vi "Load UI Config.vi"(8 "error in (no error)":errorcluster, 10 "VariableName":string, 11 "MainName":string) -> (0 "error out":errorcluster, 1 "2D Array":string[][](array[string]), 3 "1D Array":string[](array[string]), 5 "new file path (Not A Path if cancelled)":path)   [LabVIEW 2021]
uses:
  <vilib>/Utility/file.llb/Read Delimited Spreadsheet (string).vi
  <userlib>/John_Lib/TopPath/TopPath.lvlib
panel:
  out "all rows":string[][](table)
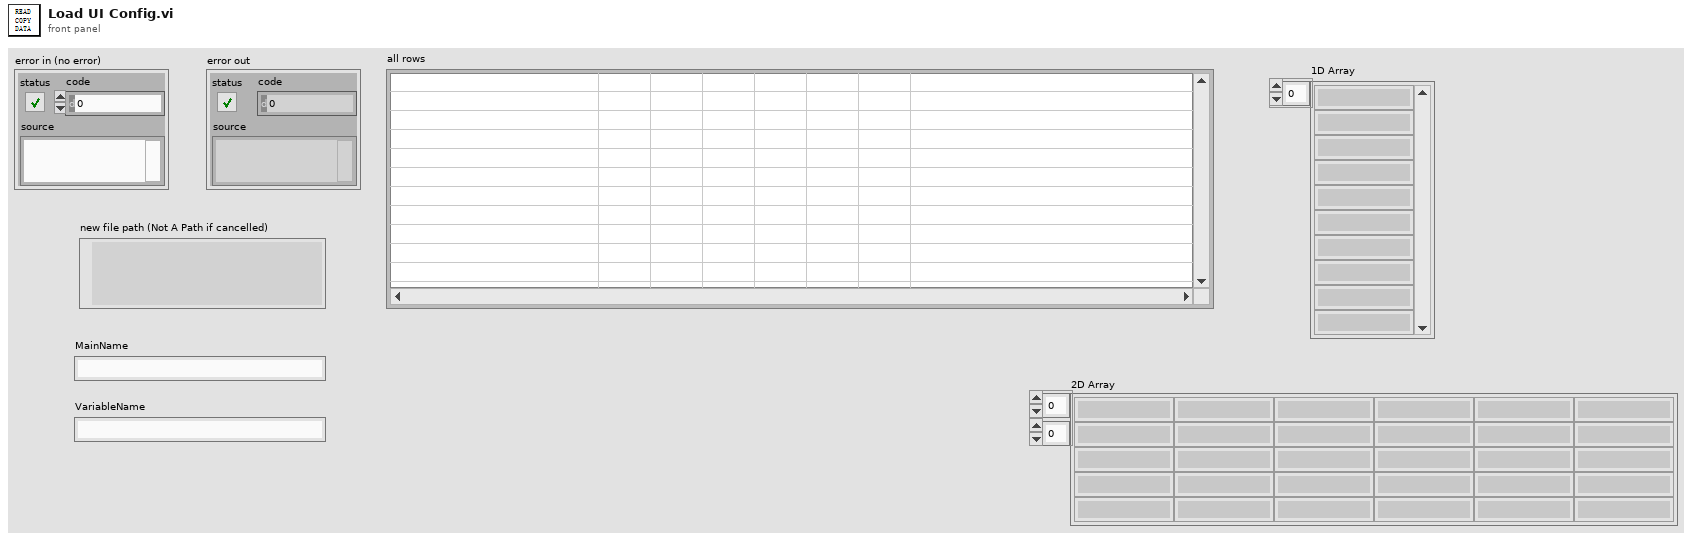
[diagram p1: front panel]
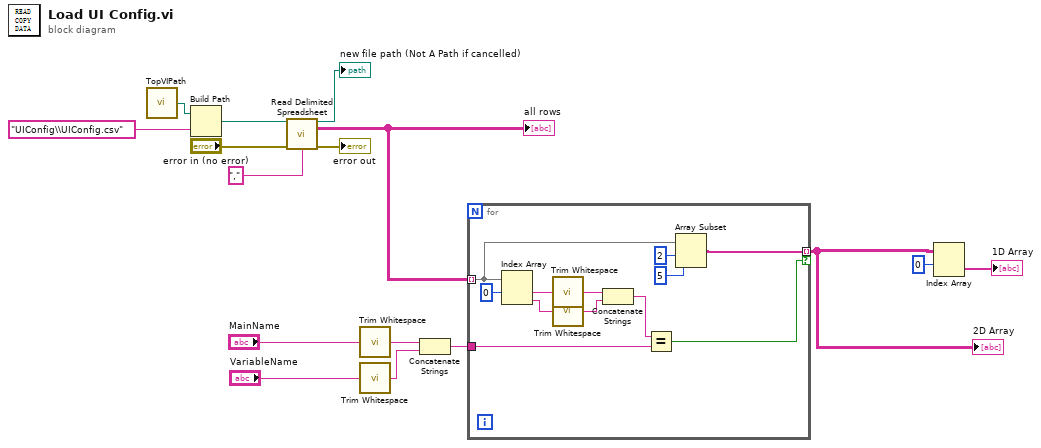
[diagram p0: block diagram]
diagram:
  n1 = call <userlib>:"TopVIPath.vi"() -> ("ConfigFile path"=w15:path)  [unwired: 2 out]
  n2 = Build Path(base path=w15, name or relative path="UIConfig\\UIConfig.csv" ("xml string")) -> (appended path=w14:path)
  n3 = call-poly <vilib>:"Read Delimited Spreadsheet.vi"("file path (dialog if empty)"=w14, "error in (no error)"="error in (no error)", "delimiter (\\t)"="," ("delimiter (\\t)")) -> ("new file path (Not A Path if cancelled)"=→"new file path (Not A Path if cancelled)":path, "all rows"=w9:string[][], "error out"=→"error out":errorcluster)  [unwired: 7 in, 3 out]
  "all rows" <- w9
  n4 = call <vilib>:"Trim Whitespace.vi"("string"="MainName") -> ("trimmed string"=w8:string)  [unwired: 1 in]
  n5 = call <vilib>:"Trim Whitespace.vi"("string"="VariableName") -> ("trimmed string"=w5:string)  [unwired: 1 in]
  n6 = Concatenate Strings(w8, w5) -> (w4:string)
  n7 = for {
    tunnel: w9 -> [w21] mode=indexing
    tunnel: w4 -> [w22]
    tunnel: [w18] -> w3 mode=indexing if=w17
    n8 = Index Array(array=w21, index #1=0 ("index")) -> (element #1=w27:string, element #2=w26:string)  [unwired: 1 in]
    n9 = call <vilib>:"Trim Whitespace.vi"("string"=w27) -> ("trimmed string"=w25:string)  [unwired: 1 in]
    n10 = call <vilib>:"Trim Whitespace.vi"("string"=w26) -> ("trimmed string"=w24:string)  [unwired: 1 in]
    n11 = Concatenate Strings(w25, w24) -> (w23:string)
    n12 = Equal?(x=w23, y=w22) -> (x = y?=w17:bool)
    n13 = Array Subset(array=w21, index=2, length=5) -> (w18:string[])
  }
  "2D Array" <- w3
  n14 = Index Array(array=w3, index (row)=0) -> (element=→"1D Array":string[])  [unwired: 1 in]
